vi "PF_PtoV.vi"(7 "Experiment Root":path, 9 "Phase":dbl[](array[numeric]), 10 "Intensity":dbl[](array[numeric]), 11 "Starting Pixel":i32) -> (1 "Mask B Voltages":dbl[](array[numeric]), 2 "Mask A Voltages":dbl[](array[numeric]))   [LabVIEW 2019]
uses:
  <vilib>/Utility/file.llb/Read Delimited Spreadsheet (DBL).vi
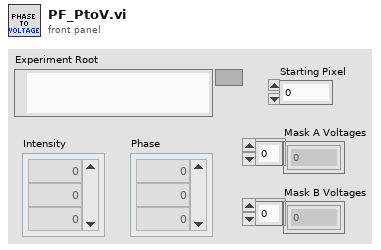
[diagram p1: front panel]
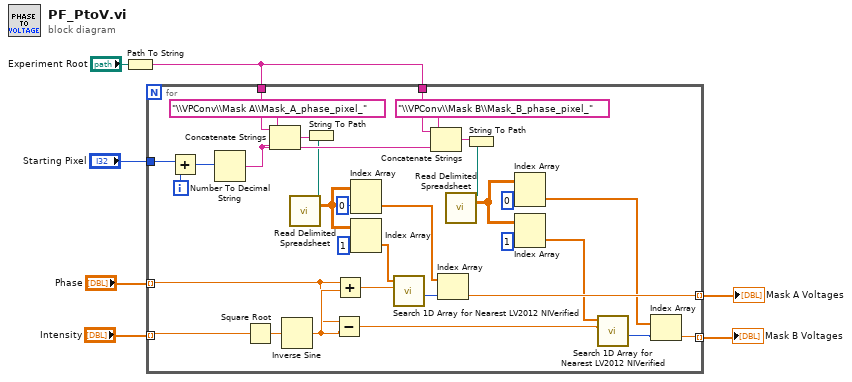
[diagram p0: block diagram]
diagram:
  n1 = Path To String(path="Experiment Root") -> (string=w4:string)
  n2 = for {
    tunnel: "Phase" -> [w36] mode=indexing
    tunnel: "Intensity" -> [w39] mode=indexing
    tunnel: [w31] -> w3 mode=indexing
    tunnel: [w30] -> w2 mode=indexing
    tunnel: w4 -> [w29]
    tunnel: w4 -> [w26]
    tunnel: "Starting Pixel" -> [w24]
    i -> [w25]
    n3 = Add(x=w24, y=w25) -> (x+y=w23:i32)
    n4 = Number To Decimal String(number=w23) -> (decimal integer string=w22:string)  [unwired: 1 in]
    n5 = Square Root(x=w39) -> (sqrt(x)=w38:dbl)
    n6 = Concatenate Strings(w29, "\\VPConv\\Mask A\\Mask_A_phase_pixel_" ("string"), w22) -> (w21:string)
    n7 = Inverse Sine(1:w38) -> (0:w37:dbl)
    n8 = String To Path(string=w21) -> (path=w19:path)
    n9 = call-poly <vilib>:"Read Delimited Spreadsheet.vi"("file path (dialog if empty)"=w19) -> ("all rows"=w16:dbl[][])  [unwired: 9 in, 5 out]
    n10 = Subtract(x=w36, y=w37) -> (x-y=w34:dbl)
    n11 = Add(x=w36, y=w37) -> (x+y=w35:dbl)
    n12 = Index Array(array=w16, index (col)=0 ("disabled index (col)")) -> (element=w10:dbl[])  [unwired: 1 in]
    n13 = Index Array(array=w16, index (col)=1 ("disabled index (col)")) -> (element=w11:dbl[])  [unwired: 1 in]
    n14 = call "Search 1D Array for Nearest LV2012 NIVerified.vi"("desired element"=w35, "1D Array"=w11) -> ("closest index"=w33:i32)  [unwired: 8 in, 1 out]
    n15 = Concatenate Strings(w26, "\\VPConv\\Mask B\\Mask_B_phase_pixel_" ("string"), w22) -> (w20:string)
    n16 = Index Array(array=w10, index=w33) -> (element=w31:dbl)
    n17 = String To Path(string=w20) -> (path=w18:path)
    n18 = call-poly <vilib>:"Read Delimited Spreadsheet.vi"("file path (dialog if empty)"=w18) -> ("all rows"=w17:dbl[][])  [unwired: 9 in, 5 out]
    n19 = Index Array(array=w17, index (col)=0 ("disabled index (col)")) -> (element=w8:dbl[])  [unwired: 1 in]
    n20 = Index Array(array=w17, index (col)=1 ("disabled index (col)")) -> (element=w9:dbl[])  [unwired: 1 in]
    n21 = call "Search 1D Array for Nearest LV2012 NIVerified.vi"("desired element"=w34, "1D Array"=w9) -> ("closest index"=w32:i32)  [unwired: 8 in, 1 out]
    n22 = Index Array(array=w8, index=w32) -> (element=w30:dbl)
  }
  "Mask A Voltages" <- w3
  "Mask B Voltages" <- w2
